vi "SMS status FGV.vi"(2 "Action":T2, 4 "PSU Status In":T1 {"Trip Current" format="%.3f"; "Trip Field" format="%.4f"; "Voltage" format="%.2f"; "Field Constant" format="%.6f"; "MID Setpoint (T)" format="%.4f"; "MID Setpoint (A)" format="%.3f"; "MAX Setpoint (T)" format="%.4f"; "MAX Setpoint (A)" format="%.3f"; "Heater Voltage" format="%.2f"; "V Limit (V)" format="%.2f"; "Ramp Rate (A/s)" format="%.3f"; "Output (A)" format="%.3f"; "Output (T)" format="%.4f"; "Persistent Current" format="%.3f"; "Persistent Field" format="%.4f"}) -> (1 "PSU status array":T1[](array[typedef]) {"Trip Current" format="%.3f"; "Trip Field" format="%.4f"; "Voltage" format="%.2f"; "Field Constant" format="%.6f"; "MID Setpoint (T)" format="%.4f"; "MID Setpoint (A)" format="%.3f"; "MAX Setpoint (T)" format="%.4f"; "MAX Setpoint (A)" format="%.3f"; "Heater Voltage" format="%.2f"; "V Limit (V)" format="%.2f"; "Ramp Rate (A/s)" format="%.3f"; "Output (A)" format="%.3f"; "Output (T)" format="%.4f"; "Persistent Current" format="%.3f"; "Persistent Field" format="%.4f"})   [LabVIEW 2017]
uses:
  <instrlib>/SMS drivers/Public/PSU Status.ctl
  ctl/FGV action.ctl
  <instrlib>/SMS drivers/Cryogenic Ltd SMSXXX.lvlib
  Magnet module.lvlib
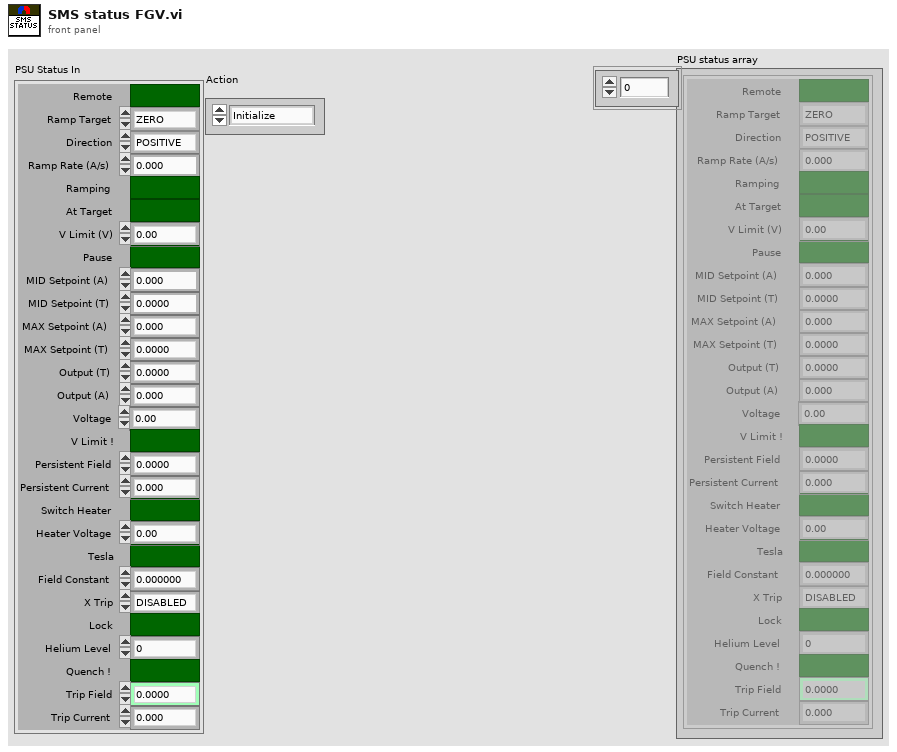
[diagram p1: front panel]
types:
  T1 = typedef "Cryogenic Ltd SMSXXX.lvlib/PSU Status.ctl" = cluster{"Ramp Target":enum16{"ZERO", "MID", "MAX"}, "Pause":bool, "Switch Heater":bool, "Persistent Field":dbl, "Persistent Current":dbl, "Tesla":bool, "Output (T)":dbl, "Output (A)":dbl, "X Trip":enum16{"DISABLED", "ENABLED", "ACTIVE"}, "Ramp Rate (A/s)":dbl, "V Limit (V)":dbl, "Heater Voltage":dbl, "MAX Setpoint (A)":dbl, "MAX Setpoint (T)":dbl, "MID Setpoint (A)":dbl, "MID Setpoint (T)":dbl, "Lock":bool, "Field Constant":dbl, "Remote":bool, "Direction":enum16{"POSITIVE", "NEGATIVE", "OPEN", "UNIPOLAR"}, "Helium Level":u16, "Quench !":bool, "Voltage":dbl, "V Limit !":bool, "Ramping":bool, "At Target":bool, "Trip Field":dbl, "Trip Current":dbl}
  T2 = typedef "Magnet module.lvlib/FGV action.ctl" = enum16{"Initialize", "Update", "Read", "Action"}
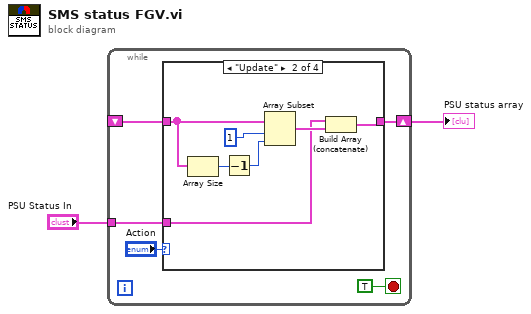
[diagram p0: block diagram]
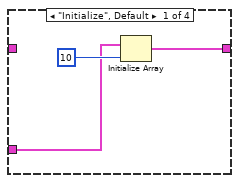
[diagram p2: hidden frame]
diagram:
  n1 = while {
    tunnel: "PSU Status In" -> [w6]
    shift-right: [w4] -> w1
    shift-left: _ -> [w3]
    stop <- TRUE stop-if-true
    n2 = case shown="\"Update\"" "Action" {
      tunnel: w6 -> [w8 w12 _ _]
      tunnel: [w9 w11 w18 w19] -> w4
      tunnel: w3 -> [_ w16 w18 w19]
      frame "Initialize", Default {
        n3 = Initialize Array(w8, 10 ("dimension size")) -> (w9:T1[])
      }
      frame "Update" {
        n4 = Array Size(array=w16) -> (size(s)=w15:i32)
        n5 = Decrement(x=w15) -> (x-1=w14:i32)
        n6 = Array Subset(array=w16, index=1, length=w14) -> (w13:T1[])
        n7 = Build Array (concatenate)(w12, w13) -> (w11:T1[])
      }
      frame "Read" {
      }
      frame "Action" {
      }
    }
  }
  "PSU status array" <- w1
